vi "SP_SetZHeights.vi"(5 "Use Overdrive?":bool, 7 "Overdrive [µm]":dbl, 8 "error in (no error)":errorcluster, 9 "Separation Distance [µm]":dbl, 10 "Contact Height [µm]":dbl, 11 "SemiProbe in":refnum<class "SemiProbe.lvclass">) -> (0 "error out":errorcluster, 3 "SemiProbe out":refnum<class "SemiProbe.lvclass">)   [LabVIEW 2018, in "SemiProbe.lvclass"]
uses:
  SemiProbe.lvclass
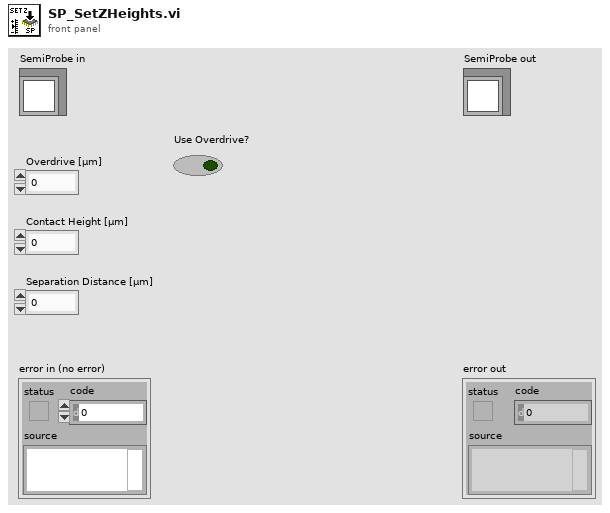
[diagram p1: front panel]
types:
  T1 = cluster{"SP Load Less Than Thr?":bool, "SP Load Threshold (um)":dbl, "SP Current Location":cluster{"X (um)":ext, "Y (um)":ext, "Z (um)":ext, "T (degree)":ext}, "SP Chuck Speeds":cluster{"XY Speed (10-100%)":dbl, "Z Speed (10-100%)":dbl, "T Speed (10-100%)":dbl}, "Manual Step Parameters":cluster{"Step in X":bool, "X S-Speed [µm/step]":sgl, "Step in Y":bool, "Y S-Speed [µm/step]":sgl, "Step in Z":bool, "Z S-Speed [µm/step]":sgl, "Step in T":bool, "T S-Speed [mdegree/step]":sgl, "X Increase":bool, "Y Increase?":bool, "Z Increase?":bool, "T Increase?":bool}, "Z Stepper":cluster{"UP/DOWN":bool, "UP/DOWN Speed [µm/step]":i32, "SP Z Step":bool}, "Z Heights Set":bool, "SP Contact Search":cluster{"Contact Circuit":enum16{"12", "1", "2"}, "Speed [1000-10000]":sgl, "Start Height [µm]":sgl, "Search Band [µm]":sgl, "Overdrive [µm]":sgl}, "Separation Distance [µm]":u32, "Contact Height [µm]":u32, "Use Overdrive?":bool, "Touchdown method":enum16{"no feedback", "Arduino edgesense", "SP contact circuit"}, "Arduino Edgesense params":cluster{"touchdown height [µm]":i32, "search band [µm]":u32, "speed [µm/step]":u32, "overdrive [µm]":u32}}
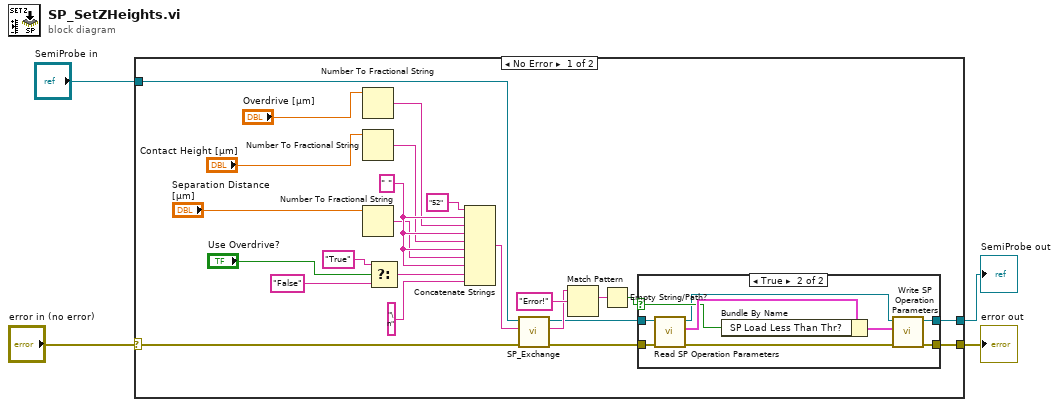
[diagram p0: block diagram]
diagram:
  n1 = case shown="No Error" "error in (no error)" {
    selector: "error in (no error)" -> [w13 w41]
    tunnel: [w6 w41] -> w3
    tunnel: [w5 w40] -> w1
    tunnel: "SemiProbe in" -> [w14 w40]
    frame No Error {
      w24 = " "
      n2 = Number To Fractional String(number="Overdrive [µm]") -> (F-format string=w23:string)  [unwired: 3 in]
      n3 = Number To Fractional String(number="Contact Height [µm]") -> (F-format string=w22:string)  [unwired: 3 in]
      n4 = Number To Fractional String(number="Separation Distance [µm]") -> (F-format string=w21:string)  [unwired: 3 in]
      n5 = Select(t="True", s="Use Overdrive?", f="False") -> (s? t:f=w16:string)
      n6 = Concatenate Strings("52", w24, w23, w24, w22, w24, w21, w24, w16, "\n") -> (w15:string)
      n7 = call-dynamic "SP_Exchange.vi"("error in (no error)"=w13, "command"=w15, "SemiProbe in"=w14) -> ("error out"=w7:errorcluster, "answer"=w11:string, "SemiProbe out"=w8:refnum<class "SemiProbe.lvclass">)  [unwired: 4 in, 2 out]
      n8 = Match Pattern(string=w11, regular expression="Error!") -> (match substring=w10:string)  [unwired: 1 in, 3 out]
      n9 = Empty String/Path?(string/path=w10) -> (empty?=w9:bool)
      n10 = case shown="True" w9 {
        selector: w9 -> [_ w34]
        tunnel: w8 -> [w30 w37]
        tunnel: w7 -> [w29 w36]
        tunnel: [w29 w39] -> w6
        tunnel: [w30 w38] -> w5
        frame False {
        }
        frame True {
          n11 = call-dynamic "Read SP Operation Parameters.vi"("error in (no error)"=w36, "SemiProbe in"=w37) -> ("error out"=w31:errorcluster, "SP Operation Parameters"=w35:T1, "SemiProbe out"=w32:refnum<class "SemiProbe.lvclass">)  [unwired: 7 in]
          n12 = Bundle By Name(cluster=w35, "SP Load Less Than Thr?"=w34) -> (w33:T1)
          n13 = call-dynamic "Write SP Operation Parameters.vi"("error in (no error)"=w31, "SP Operation Parameters"=w33, "SemiProbe in"=w32) -> ("error out"=w39:errorcluster, "SemiProbe out"=w38:refnum<class "SemiProbe.lvclass">)  [unwired: 7 in]
        }
      }
    }
    frame Error {
    }
  }
  "error out" <- w3
  "SemiProbe out" <- w1
